vi "gRPC Client Test.vi"(8 "error in":errorcluster, 9 "CI.Freq.MeasTime in":dbl, 10 "counter":tag, 11 "task name":string) -> (0 "error out":errorcluster, 3 "CI.Freq.MeasTime out":dbl)   [LabVIEW 2021, in "NI_DAQmx_client.lvlib"]
uses:
  NI_DAQmx_client.lvlib
  <vilib>/Plug-In SDKs/Measurements/Measure Call Context/Measure Call Context.lvclass
  Session Factory/Client Wrapper Functions/niDAQmx gRPC Device Server.ctl
  Session Factory/Session Factory.lvclass
  Session Management niDAQmx.lvlib
  <vilib>/Plug-In SDKs/Clients/Session Management V1/Session Reservation/Initialize and Close Session Behavior.ctl
  <vilib>/Plug-In SDKs/Clients/Session Management V1/Session Reservation/Session Reservation.lvclass
  Initialize Tasks - 1Task.vi
  <vilib>/Plug-In SDKs/Measurements/Measure Call Context/Reserve Sessions - 1Pin.vi
panel:
  out "error out 3":errorcluster
  out "CI.Freq.MeasTime out 2":dbl
  in  "error in 3":errorcluster
  in  "task name 2":string
  out "error out 2":errorcluster
  in  "CI.Freq.MeasTime in 2":dbl
  in  "counter 2":tag
  out "measurement context out":refnum<class "Measure Call Context.lvclass">
  in  "error in 2":errorcluster
  in  "pin or relay name":string
  in  "measurement context in":refnum<class "Measure Call Context.lvclass">
  # "Example in Disabled Structure"
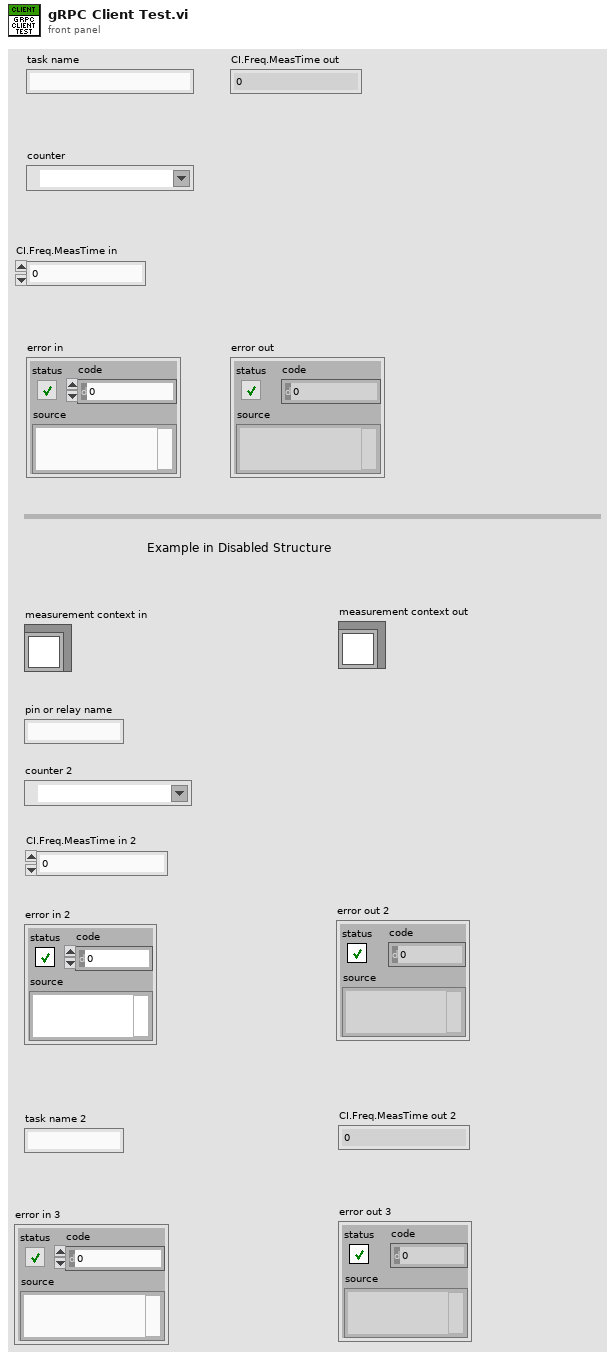
[diagram p1: front panel]
types:
  T1 = typedef "Session Management niDAQmx.lvlib/Session Factory.lvclass/niDAQmx gRPC Device Server.ctl" = cluster{"task name":string, "address (localhost)":string, "port (31763)":u32}
  T2 = typedef "NI Session Management V1 Client.lvlib/Session Reservation.lvclass/Initialize and Close Session Behavior.ctl" = enum16{"Auto", "Initialize and Close", "Attach and Detach", "Initialize and Detach", "Attach and Close"}
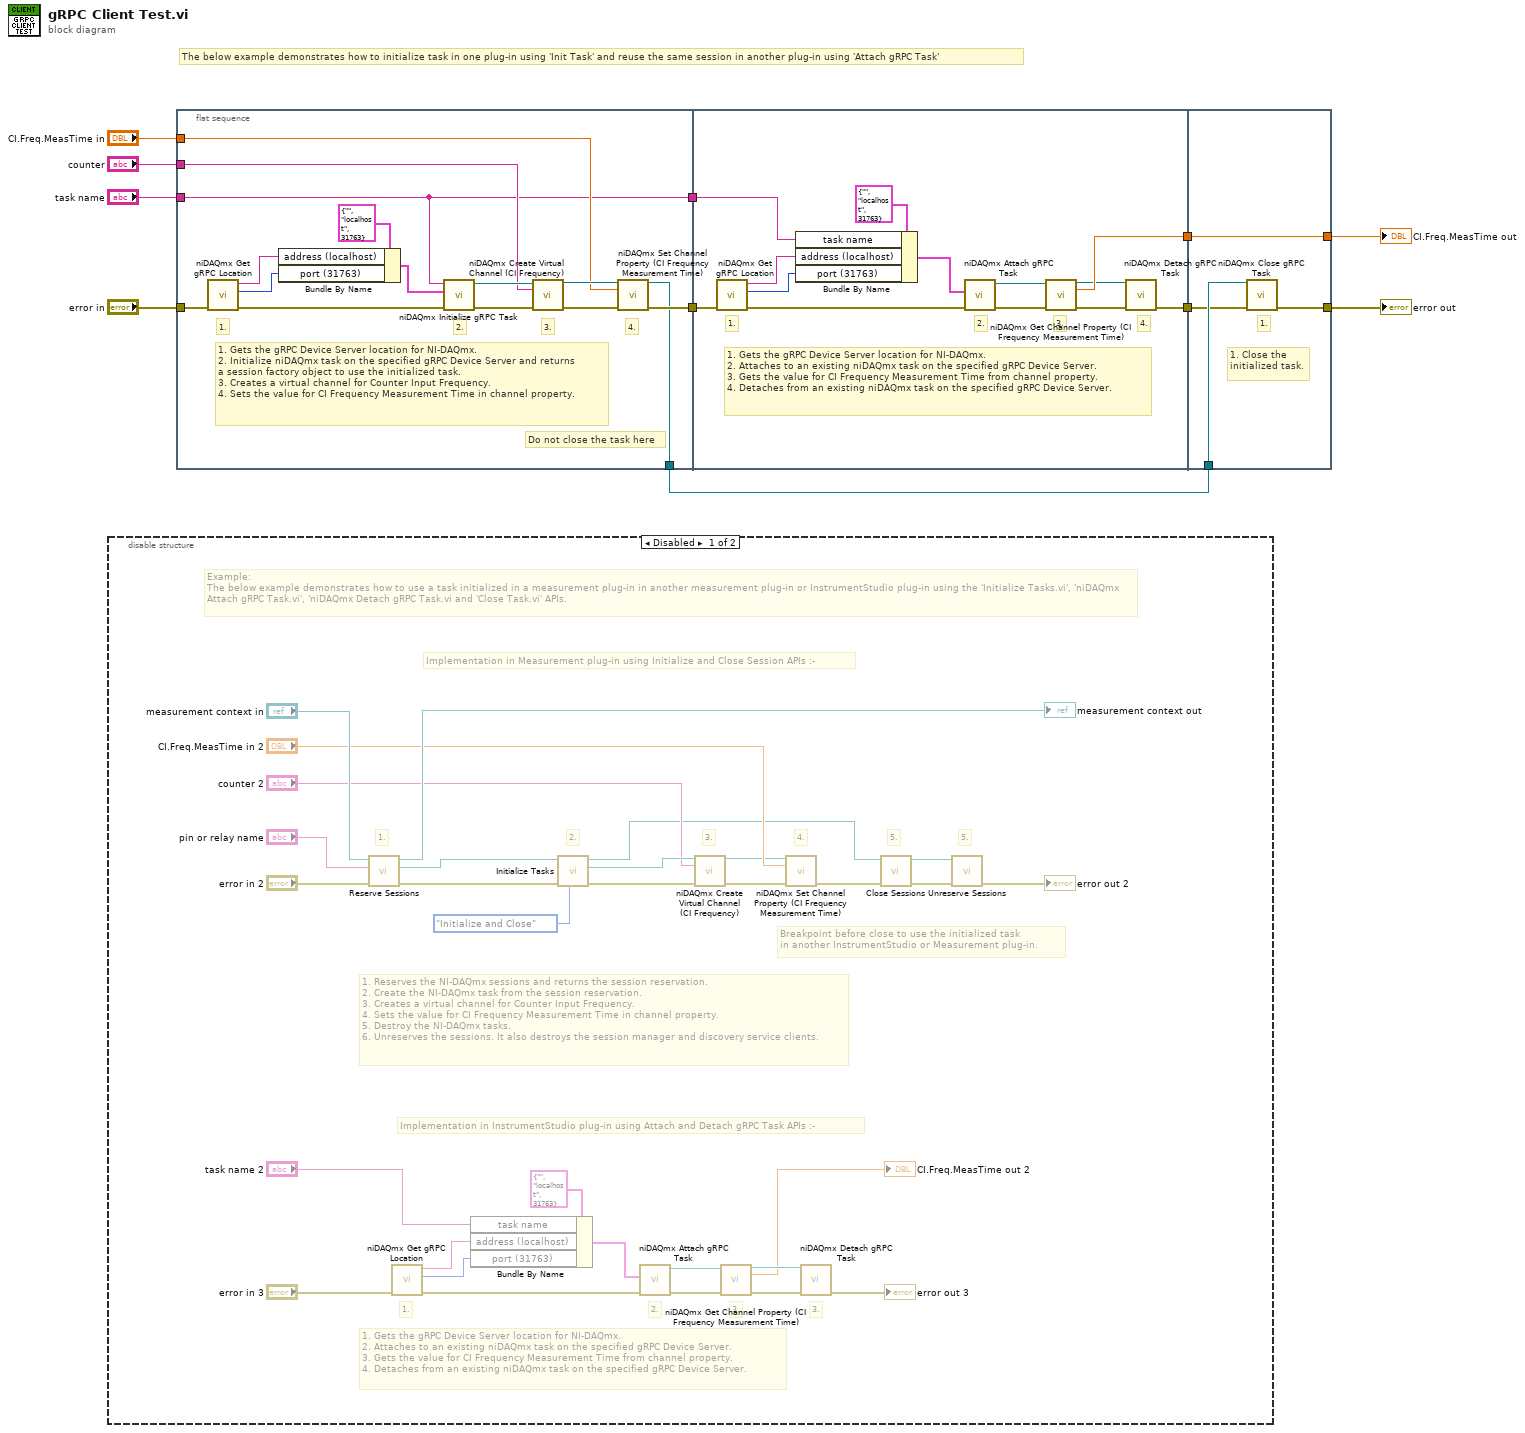
[diagram p0: block diagram]
diagram:
  # "The below example demonstrates how to initialize task in one plug-in using 'Init Task' and reuse the same session in another plug-in using 'Attach gRPC Task'"
  n1 = disable-structure shown="Disabled" {
    frame Disabled {
      # "3."
      # "3."
      # "2."
      # "1."
      # "1. Gets the gRPC Device Server location for NI-DAQmx.\n2. Attaches to an existing niDAQmx task on the specified gRPC Device Server.\n3. Gets the value for CI Frequency Measurement Time from channel property.\n4. Detaches from an existing niDAQmx task on the specified gRPC Device Server."
      # "1. Reserves the NI-DAQmx sessions and returns the session reservation.\n2. Create the NI-DAQmx task from the session reservation.\n3. Creates a virtual channel for Counter Input Frequency. \n4. Sets the value for CI Frequency Measurement Time in channel property. \n5. Destroy the NI-DAQmx tasks.\n6. Unreserves the sessions. It also destroys the session manager and discovery service clients."
      # "5."
      # "5."
      # "4."
      # "3."
      # "2."
      # "1."
      # "Implementation in InstrumentStudio plug-in using Attach and Detach gRPC Task APIs :-"
      # "Breakpoint before close to use the initialized task\nin another InstrumentStudio or Measurement plug-in."
      # "Implementation in Measurement plug-in using Initialize and Close Session APIs :-"
      # "Example:\nThe below example demonstrates how to use a task initialized in a measurement plug-in in another measurement plug-in or InstrumentStudio plug-in using the 'Initialize Tasks.vi', 'niDAQmx Attach gRPC Task.vi', 'niDAQmx Detach gRPC Task.vi and 'Close Task.vi' APIs."
      n2 = call-poly <vilib>:"Reserve Sessions.vi"("error in"="error in 2", "pin or relay name"="pin or relay name", "measurement context in"="measurement context in") -> ("error out"=w39:errorcluster, "session reservation out"=w37:refnum<class "Session Reservation.lvclass">, "measurement context out"=→"measurement context out":refnum<class "Measure Call Context.lvclass">)  [unwired: 6 in]
      n3 = call "niDAQmx Get gRPC Location.vi"("error in"="error in 3") -> ("error out"=w21:errorcluster, "port"=w22:u32, "address"=w23:string)  [unwired: 8 in]
      n4 = Bundle By Name(cluster=T1 {"task name"="", "address (localhost)"="localhost", "port (31763)"=31763} ("gRPC options"), "task name"="task name 2", "address (localhost)"=w23, "port (31763)"=w22) -> (w20:T1)
      n5 = call-poly "Initialize Tasks.vi"("initialize and close session behavior"=Initialize_and_Close_Session_Behavior."Initialize and Close", "error in"=w39, "session reservation in"=w37) -> ("error out"=w35:errorcluster, "task"=w34:refnum<class "Session Factory.lvclass">, "session reservation out"=w26:refnum<class "Session Reservation.lvclass">)  [unwired: 5 in, 1 out]
      n6 = call "niDAQmx Attach gRPC Task.vi"("error in"=w21, "gRPC options"=w20) -> ("error out"=w19:errorcluster, "task out"=w18:refnum<class "Session Factory.lvclass">)  [unwired: 8 in]
      n7 = call "niDAQmx Create Virtual Channel (CI Frequency).vi"("task in"=w34, "counter"="counter 2", "error in"=w35) -> ("task out"=w30:refnum<class "Session Factory.lvclass">, "error out"=w32:errorcluster)  [unwired: 11 in]
      n8 = call "niDAQmx Get Channel Property (CI Frequency Measurement Time).vi"("task in"=w18, "error in"=w19) -> ("task out"=w16:refnum<class "Session Factory.lvclass">, "CI.Freq.MeasTime"=→"CI.Freq.MeasTime out 2":dbl, "error out"=w17:errorcluster)  [unwired: 11 in]
      n9 = call "niDAQmx Set Channel Property (CI Frequency Measurement Time).vi"("task in"=w30, "CI.Freq.MeasTime"="CI.Freq.MeasTime in 2", "error in"=w32) -> ("error out"=w28:errorcluster)  [unwired: 11 in, 1 out]
      n10 = call "niDAQmx Detach gRPC Task.vi"("task in"=w16, "error in"=w17) -> ("error out"=→"error out 3":errorcluster)  [unwired: 13 in]
      n11 = call <vilib>:"Close Sessions.vi"("error in"=w28, "session reservation in"=w26) -> ("error out"=w27:errorcluster, "session reservation out"=w29:refnum<class "Session Reservation.lvclass">)  [unwired: 8 in]
      n12 = call <vilib>:"Unreserve Sessions.vi"("error in"=w27, "session reservation in"=w29) -> ("error out"=→"error out 2":errorcluster)  [unwired: 9 in]
    }
    frame Enabled {
    }
  }
  n13 = flat-sequence {
    tunnel: "error in" -> [w57]
    tunnel: "task name" -> [w43]
    tunnel: "counter" -> [w49]
    tunnel: "CI.Freq.MeasTime in" -> [w46]
    tunnel: [w45] -> w7
    tunnel: [w44] -> w2
    tunnel: [w43] -> w6
    tunnel: w7 -> [w67]
    tunnel: w6 -> [w64]
    tunnel: [w60] -> w5
    tunnel: [w58] -> w3
    tunnel: [w74] -> w4
    tunnel: w5 -> [w74]
    tunnel: w3 -> [w71]
    tunnel: [w72] -> w1
    tunnel: w2 -> [w73]
    frame #0 {
      # "Do not close the task here"
      # "1. Gets the gRPC Device Server location for NI-DAQmx.\n2. Initialize niDAQmx task on the specified gRPC Device Server and returns\na session factory object to use the initialized task.\n3. Creates a virtual channel for Counter Input Frequency.\n4. Sets the value for CI Frequency Measurement Time in channel property."
      # "4."
      # "3."
      # "2."
      # "1."
      n14 = call "niDAQmx Get gRPC Location.vi"("error in"=w57) -> ("error out"=w52:errorcluster, "port"=w54:u32, "address"=w55:string)  [unwired: 8 in]
      n15 = Bundle By Name(cluster=T1 {"task name"="", "address (localhost)"="localhost", "port (31763)"=31763} ("gRPC options"), "address (localhost)"=w55, "port (31763)"=w54) -> (w53:T1)
      n16 = call "niDAQmx Initialize gRPC Task.vi"("error in"=w52, "gRPC options"=w53, "task name"=w43) -> ("error out"=w51:errorcluster, "task out"=w50:refnum<class "Session Factory.lvclass">)  [unwired: 7 in]
      n17 = call "niDAQmx Create Virtual Channel (CI Frequency).vi"("task in"=w50, "counter"=w49, "error in"=w51) -> ("task out"=w47:refnum<class "Session Factory.lvclass">, "error out"=w48:errorcluster)  [unwired: 11 in]
      n18 = call "niDAQmx Set Channel Property (CI Frequency Measurement Time).vi"("task in"=w47, "CI.Freq.MeasTime"=w46, "error in"=w48) -> ("task out"=w44:refnum<class "Session Factory.lvclass">, "error out"=w45:errorcluster)  [unwired: 11 in]
    }
    frame #1 {
      # "4."
      # "3."
      # "2."
      # "1."
      # "1. Gets the gRPC Device Server location for NI-DAQmx.\n2. Attaches to an existing niDAQmx task on the specified gRPC Device Server.\n3. Gets the value for CI Frequency Measurement Time from channel property.\n4. Detaches from an existing niDAQmx task on the specified gRPC Device Server."
      n19 = call "niDAQmx Get gRPC Location.vi"("error in"=w67) -> ("error out"=w66:errorcluster, "port"=w68:u32, "address"=w69:string)  [unwired: 8 in]
      n20 = Bundle By Name(cluster=T1 {"task name"="", "address (localhost)"="localhost", "port (31763)"=31763} ("gRPC options"), "task name"=w64, "address (localhost)"=w69, "port (31763)"=w68) -> (w65:T1)
      n21 = call "niDAQmx Attach gRPC Task.vi"("error in"=w66, "gRPC options"=w65) -> ("error out"=w63:errorcluster, "task out"=w62:refnum<class "Session Factory.lvclass">)  [unwired: 8 in]
      n22 = call "niDAQmx Get Channel Property (CI Frequency Measurement Time).vi"("task in"=w62, "error in"=w63) -> ("task out"=w59:refnum<class "Session Factory.lvclass">, "CI.Freq.MeasTime"=w60:dbl, "error out"=w61:errorcluster)  [unwired: 11 in]
      n23 = call "niDAQmx Detach gRPC Task.vi"("task in"=w59, "error in"=w61) -> ("error out"=w58:errorcluster)  [unwired: 13 in]
    }
    frame #2 {
      # "1."
      # "1. Close the initialized task."
      n24 = call "niDAQmx Close gRPC Task.vi"("task in"=w73, "error in"=w71) -> ("error out"=w72:errorcluster)  [unwired: 13 in]
    }
  }
  "CI.Freq.MeasTime out" <- w4
  "error out" <- w1
